vi "Read Arm.vi"(8 "error in (no error)":errorcluster, 11 "Fault-Insertion_Value in":refnum<class "Fault-Insertion_Type.lvclass">) -> (0 "error out":errorcluster, 2 "Armed?":bool, 3 "Fault-Insertion_Value out":refnum<class "Fault-Insertion_Type.lvclass">)   [LabVIEW 2021, in "Fault-Insertion_Type.lvclass"]
uses:
  Fault-Insertion_Type.lvclass
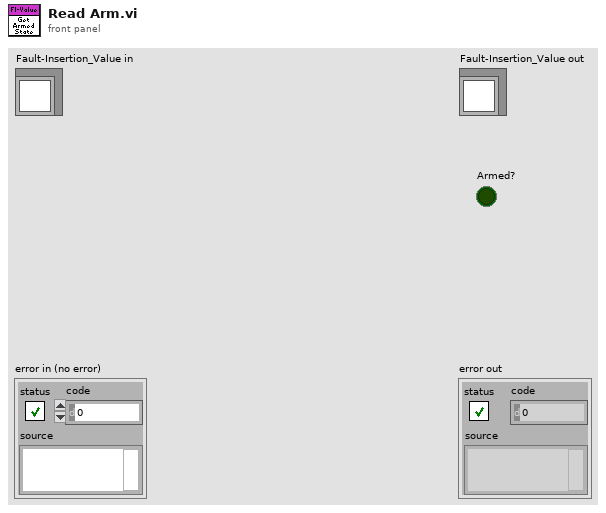
[diagram p1: front panel]
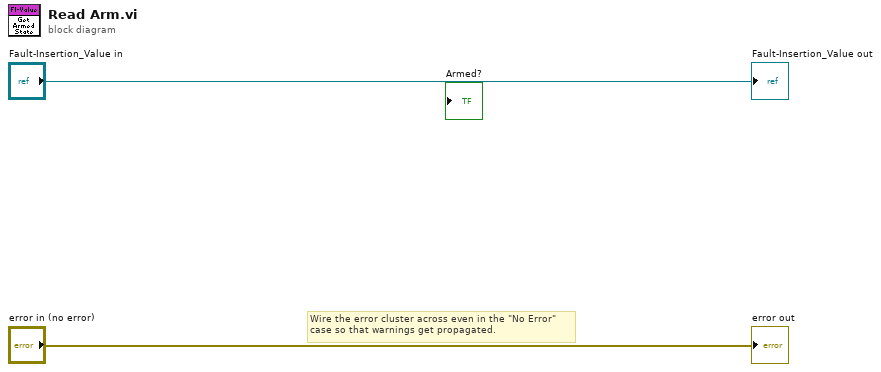
[diagram p0: block diagram]
diagram:
  # "Wire the error cluster across even in the \"No Error\"\ncase so that warnings get propagated."
  "error out" <- "error in (no error)"
  "Fault-Insertion_Value out" <- "Fault-Insertion_Value in"
